vi "Eol Exc Time.vi"(8 "error in (no error)":errorcluster, 10 "Mode":string[](array[string]), 11 "base":path) -> (0 "error out":errorcluster, 2 "Array":timestamp[](array[timestamp]), 3 "Numeric":dbl)   [LabVIEW 2014]
uses:
  <vilib>/Utility/file.llb/Read Delimited Spreadsheet (string).vi
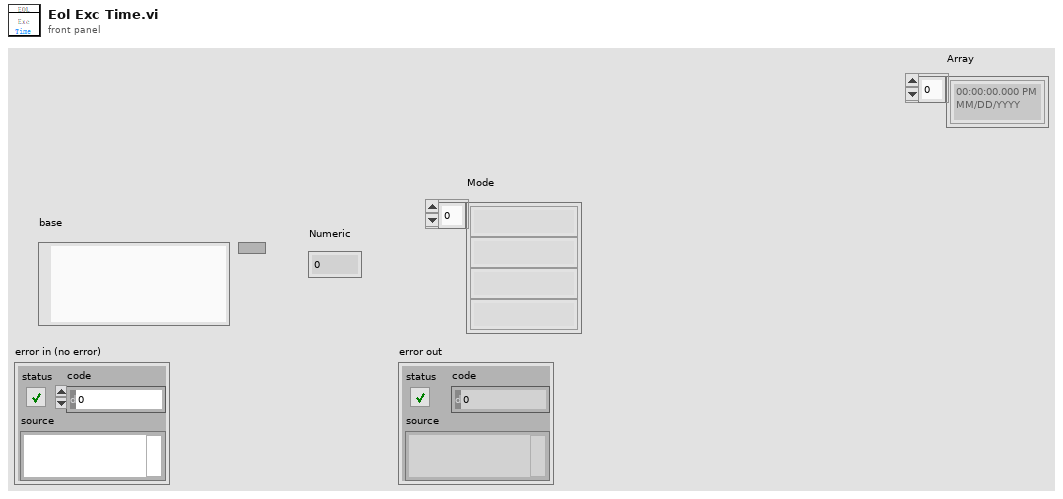
[diagram p1: front panel]
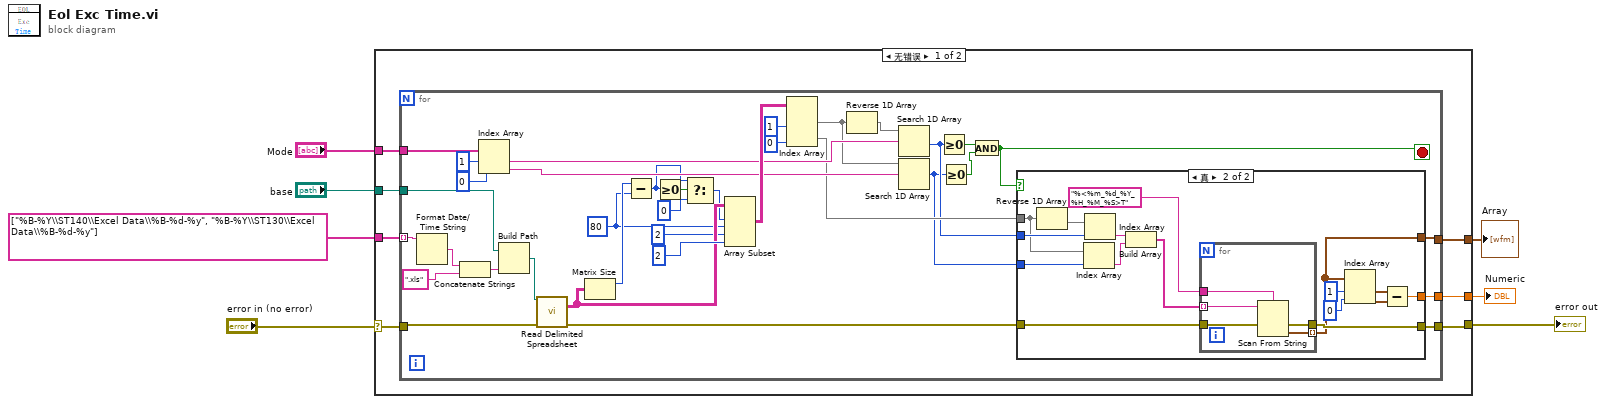
[diagram p0: block diagram]
diagram:
  n1 = case shown="无错误" "error in (no error)" {
    selector: "error in (no error)" -> [w14 w73]
    tunnel: "base" -> [w12 _]
    tunnel: string[] ["%B-%Y\\ST140\\Excel Data\\%B-%d-%y", "%B-%Y\\ST130\\Excel Data\\%B-%d-%y"] -> [w13 _]
    tunnel: "Mode" -> [w11 _]
    tunnel: [w10 _] -> w3
    tunnel: [w9 w73] -> w2
    tunnel: [w8 _] -> w1
    frame No Error {
      n2 = for {
        tunnel: w14 -> [w45]
        tunnel: w13 -> [w50] mode=indexing
        tunnel: w12 -> [w46]
        tunnel: w11 -> [w43]
        tunnel: [w26] -> w10
        tunnel: [w25] -> w9
        tunnel: [w15] -> w8
        stop <- w31 stop-if-true
        w21 = 80 ("length")
        n3 = Format Date/Time String(time format string (%c)=w50) -> (date/time string=w49:string)  [unwired: 2 in]
        n4 = Concatenate Strings(w49, ".xls" ("string")) -> (w47:string)
        n5 = Index Array(array=w43, index #1=1 ("index"), index #2=0 ("index")) -> (element #1=w38:string, element #2=w35:string)
        n6 = Build Path(base path=w46, name or relative path=w47) -> (appended path=w16:path)
        n7 = call-poly <vilib>:"Read Delimited Spreadsheet.vi"("file path (dialog if empty)"=w16, "error in (no error)"=w45) -> ("all rows"=w24:string[][], "error out"=w27:errorcluster)  [unwired: 8 in, 4 out]
        n8 = Matrix Size(0:w24) -> (1:w22:i32)  [unwired: 1 out]
        n9 = Subtract(x=w22, y=w21) -> (x-y=w19:i32)
        n10 = Greater Or Equal To 0?(x=w19) -> (x >= 0?=w20:bool)
        n11 = Select(t=w19, s=w20, f=0) -> (s? t:f=w18:i32)
        n12 = Array Subset(array=w24, index (row)=w18, length (row)=w21, index (col)=2 ("disabled index (col)"), length (col)=2 ("length")) -> (w40:string[][])
        n13 = Index Array(array=w40, index (col) #1=1 ("disabled index (col)"), index (col) #2=0 ("index (col)")) -> (element #1=w36:string[], element #2=w30:string[])  [unwired: 2 in]
        n14 = Reverse 1D Array(array=w36) -> (reversed array=w37:string[])
        n15 = Search 1D Array(1D array=w37, element=w38) -> (index of element=w29:i32)  [unwired: 1 in]
        n16 = Search 1D Array(1D array=w36, element=w35) -> (index of element=w28:i32)  [unwired: 1 in]
        n17 = Greater Or Equal To 0?(x=w29) -> (x >= 0?=w34:bool)
        n18 = Greater Or Equal To 0?(x=w28) -> (x >= 0?=w33:bool)
        n19 = And(x=w34, y=w33) -> (x .and. y?=w31:bool)
        n20 = case shown="真" w31 {
          tunnel: w30 -> [_ w65]
          tunnel: w29 -> [_ w66]
          tunnel: w28 -> [_ w64]
          tunnel: w27 -> [w51 w61]
          tunnel: [_ w55] -> w26
          tunnel: [w51 w54] -> w25
          tunnel: [_ w52] -> w15
          frame False {
          }
          frame True {
            n21 = Reverse 1D Array(array=w65) -> (reversed array=w67:string[])
            n22 = Index Array(array=w65, index=w64) -> (element=w62:string)
            n23 = Index Array(array=w67, index=w66) -> (element=w63:string)
            n24 = Build Array(w63, w62) -> (w53:string[])
            n25 = for {
              tunnel: w61 -> [w72]
              tunnel: "%<%m_%d_%Y_%H_%M_%S>T" ("format string") -> [w71]
              tunnel: w53 -> [w70] mode=indexing
              tunnel: [w69] -> w52 mode=indexing
              tunnel: [w68] -> w54
              n26 = Scan From String(format string=w71, input string=w70, error in=w72) -> (error out=w68:errorcluster, output 1=w69:timestamp)  [unwired: 2 in, 2 out]
            }
            n27 = Index Array(array=w52, index #1=1 ("index"), index #2=0 ("index")) -> (element #1=w56:timestamp, element #2=w57:timestamp)
            n28 = Subtract(x=w56, y=w57) -> (x-y=w55:dbl)
          }
        }
      }
    }
    frame Error {
    }
  }
  "error out" <- w2
  "Numeric" <- w3
  "Array" <- w1
